vi "SessionManager.vi"() -> ()   [LabVIEW 2014]
uses:
  TimeStamper/TimeStamper.lvclass
panel:
  in  "Bus System":string(combo)="PXI"
  in  "Acquisition System":string(combo)="NI"
  out "Stopped":bool
  out "Messages":T1(array[cluster])
  out "Timestamps":T2(array[cluster])
  out "error out":errorcluster
  in  "Experimenter":string(combo)="Unselected"
  out "Session Path":path
  in  "stop":bool
  in  "Subject":string(combo)="Testing"
  in  "Counter Card":tag="Dev1"
  in  "Sample Lines":tag[](array[tag])=["/Dev3/ai/StartTrigger", "/Dev1/PXI_Trig4", "/4498_1/ai/StartTrigger", "/Dev1/PXI_Trig5", "/Dev1/PFI8"]
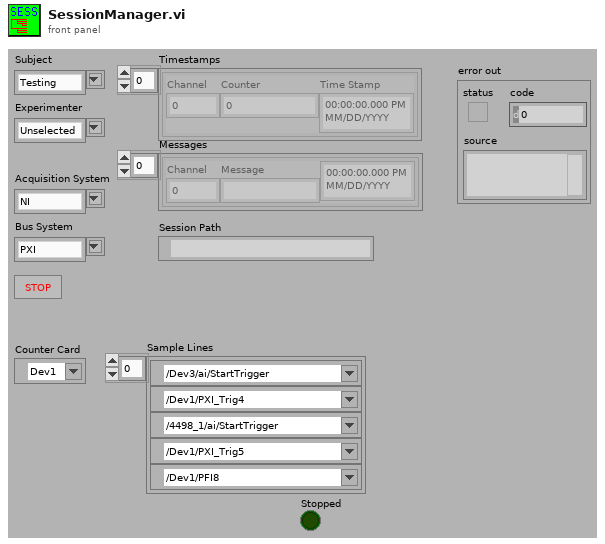
[diagram p1: front panel]
types:
  T1 = cluster{"Channel":dbl, "Message":string, timestamp}[]
  T2 = cluster{"Channel":i32, "Counter":u32, "Time Stamp":timestamp}[]
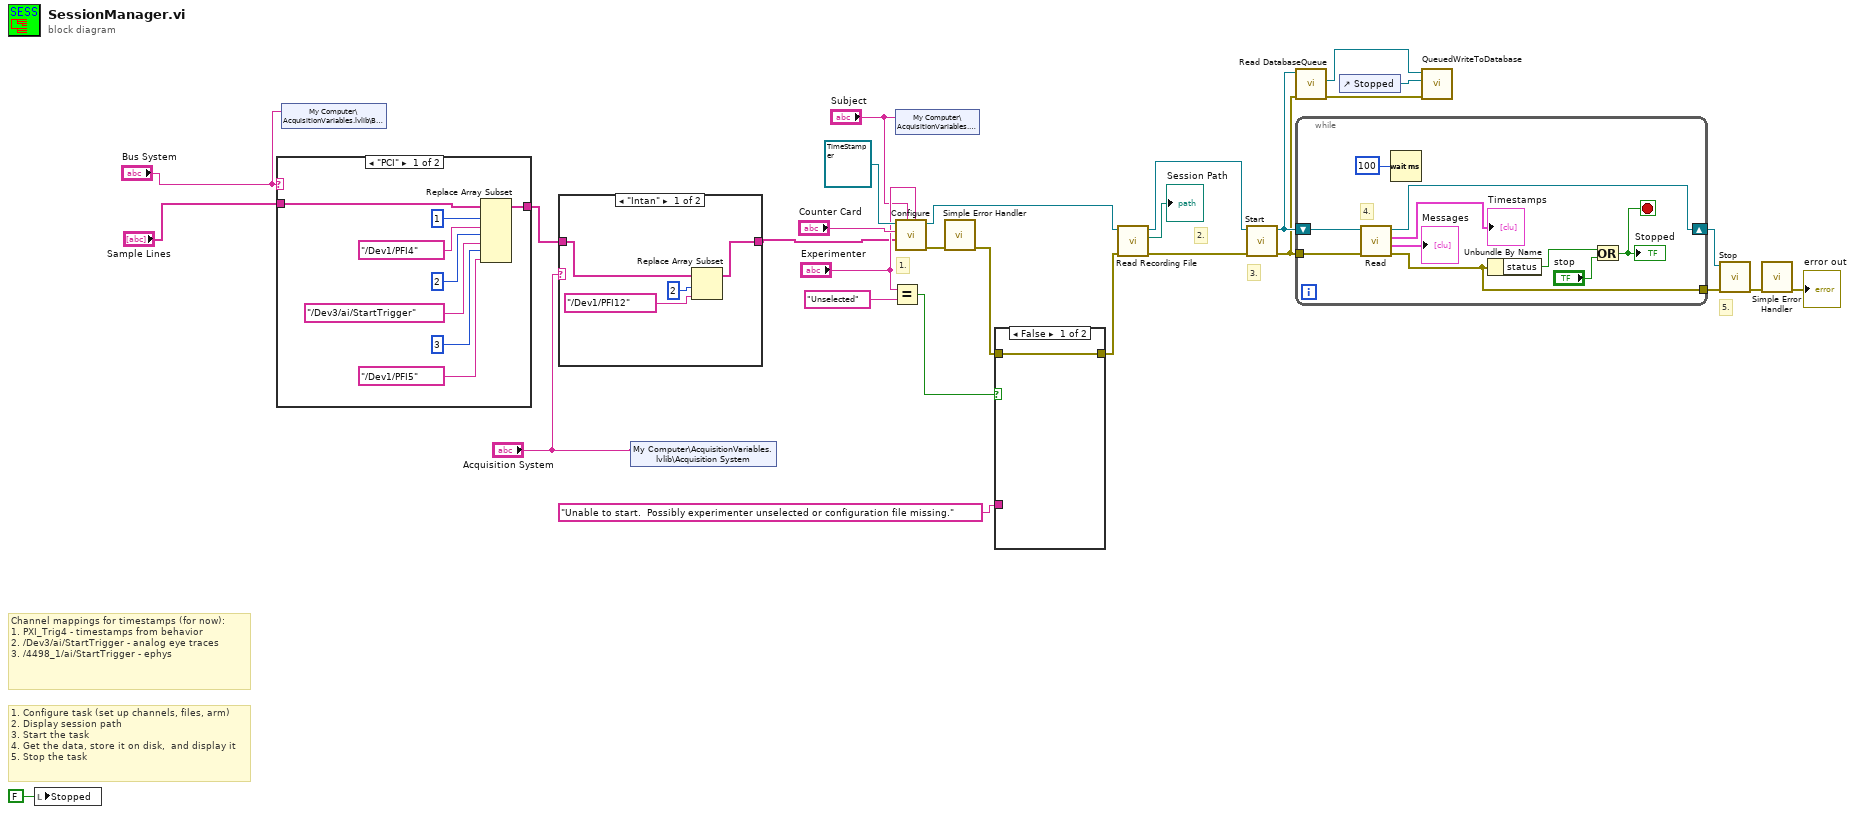
[diagram p0: block diagram]
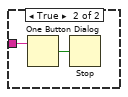
[diagram p4: hidden frame]
diagram:
  # "Channel mappings for timestamps (for now):\n1. PXI_Trig4 - timestamps from behavior\n2. /Dev3/ai/StartTrigger - analog eye traces\n3. /4498_1/ai/StartTrigger - ephys"
  # "1. Configure task (set up channels, files, arm)\n2. Display session path\n3. Start the task\n4. Get the data, store it on disk,  and display it\n5. Stop the task"
  # "2."
  # "5."
  # "3."
  # "1."
  n1 = local write "Stopped"(FALSE ("Stopped")) -> ()
  n2 = case shown="\"PCI\"" "Bus System" {
    tunnel: "Sample Lines" -> [w35 w38]
    tunnel: [w34 w38] -> w3
    frame "PCI" {
      n3 = Replace Array Subset(array=w35, new element #1=tag "/Dev1/PFI4" ("new element/subarray"), index #1=1 ("index"), new element #2=tag "/Dev3/ai/StartTrigger", index #2=2 ("index"), new element #3=tag "/Dev1/PFI5" ("new element/subarray"), index #3=3 ("index")) -> (w34:tag[])
    }
    frame "PXI", Default {
    }
  }
  n4 = shared-variable "My Computer\\AcquisitionVariables.lvlib\\Bus System"("Bus System") -> ()  [unwired: 1 in, 1 out]
  n5 = case shown="\"Intan\"" "Acquisition System" {
    tunnel: w3 -> [w40 w43]
    tunnel: [w39 w43] -> w1
    frame "Intan" {
      n6 = Replace Array Subset(array=w40, new element=tag "/Dev1/PFI12" ("new element/subarray"), index=2) -> (w39:tag[])
    }
    frame "NI", Default {
    }
  }
  n7 = shared-variable "My Computer\\AcquisitionVariables.lvlib\\Acquisition System"("Acquisition System") -> ()  [unwired: 1 in, 1 out]
  n8 = Equal?(x="Experimenter", y="Unselected") -> (x = y?=w15:bool)
  n9 = shared-variable "My Computer\\AcquisitionVariables.lvlib\\Subject"("Subject") -> ()  [unwired: 1 in, 1 out]
  n10 = call-dynamic "Configure.vi"("Experimenter"="Experimenter", "Subject"="Subject", "Sample Lines"=w1, "DAQmx Device Name"="Counter Card", "TimeStamper in"=refnum<class "TimeStamper.lvclass"> refnum ("TimeStamper.lvclass")) -> ("error out"=w14:errorcluster, "TimeStamper out"=w22:refnum<class "TimeStamper.lvclass">)  [unwired: 5 in]
  n11 = call <vilib>:"Simple Error Handler.vi"("error in (no error)"=w14) -> ("error out"=w13:errorcluster)  [unwired: 4 in, 4 out]
  n12 = case shown="False" w15 {
    tunnel: "Unable to start.  Possibly experimenter unselected or configuration file missing." -> [_ w46]
    tunnel: w13 -> [w44 _]
    tunnel: [w44 _] -> w21
    frame False {
    }
    frame True {
      n13 = One Button Dialog(message=w46) -> (true=w45:bool)  [unwired: 1 in]
      n14 = Stop(stop? (T)=w45) -> ()
    }
  }
  n15 = call-dynamic "Read Recording File.vi"("error in (no error)"=w21, "AcquistionObject in"=w22) -> ("error out"=w18:errorcluster, "Recording File"=→"Session Path":path, "AcquistionObject out"=w19:refnum<class "TimeStamper.lvclass">)  [unwired: 7 in]
  n16 = call-dynamic "Start.vi"("error in (no error)"=w18, "TimeStamper in"=w19) -> ("error out"=w9:errorcluster, "TimeStamper out"=w10:refnum<class "TimeStamper.lvclass">)  [unwired: 8 in]
  n17 = call-dynamic "Read DatabaseQueue.vi"("error in (no error)"=w9, "AcquistionObject in"=w10) -> ("error out"=w7:errorcluster, "DatabaseQueue"=w8:refnum<queue>)  [unwired: 7 in, 1 out]
  n18 = while {
    tunnel: w9 -> [w54]
    shift-right: [w52] -> w28
    shift-left: w10 -> [w53]
    tunnel: [w50] -> w27
    stop <- w47 stop-if-true
    # "4."
    n19 = call-dynamic "Read.vi"("error in (no error)"=w54, "TimeStamper in"=w53) -> ("error out"=w50:errorcluster, "Messages"=→"Messages":T1, "Timestamps"=→"Timestamps":T2, "TimeStamper out"=w52:refnum<class "TimeStamper.lvclass">)  [unwired: 6 in]
    n20 = Wait (ms)(milliseconds to wait=u32 100) -> ()  [unwired: 1 out]
    n21 = Unbundle By Name(w50) -> ("status"=w49:bool)
    n22 = Or(x=w49, y="stop") -> (x .or. y?=w47:bool)
    "Stopped" <- w47
  }
  n23 = control-ref of="Stopped"() -> (w6:refnum<vi>)
  n24 = call "QueuedWriteToDatabase.vi"("error in"=w7, "Stop Flag Reference"=w6, "queue"=w8) -> ()  [unwired: 8 in, 1 out]
  n25 = call-dynamic "Stop.vi"("error in (no error)"=w27, "TimeStamper in"=w28) -> ("error out"=w11:errorcluster)  [unwired: 8 in, 1 out]
  n26 = call <vilib>:"Simple Error Handler.vi"("error in (no error)"=w11) -> ("error out"=→"error out":errorcluster)  [unwired: 4 in, 4 out]
